vi "InitControlls.vi"(8 "error in (no error)":errorcluster, 11 "Common Refs":T1) -> (0 "error out":errorcluster)   [LabVIEW 2018]
uses:
  TypeDefs/Refs_Common.ctl
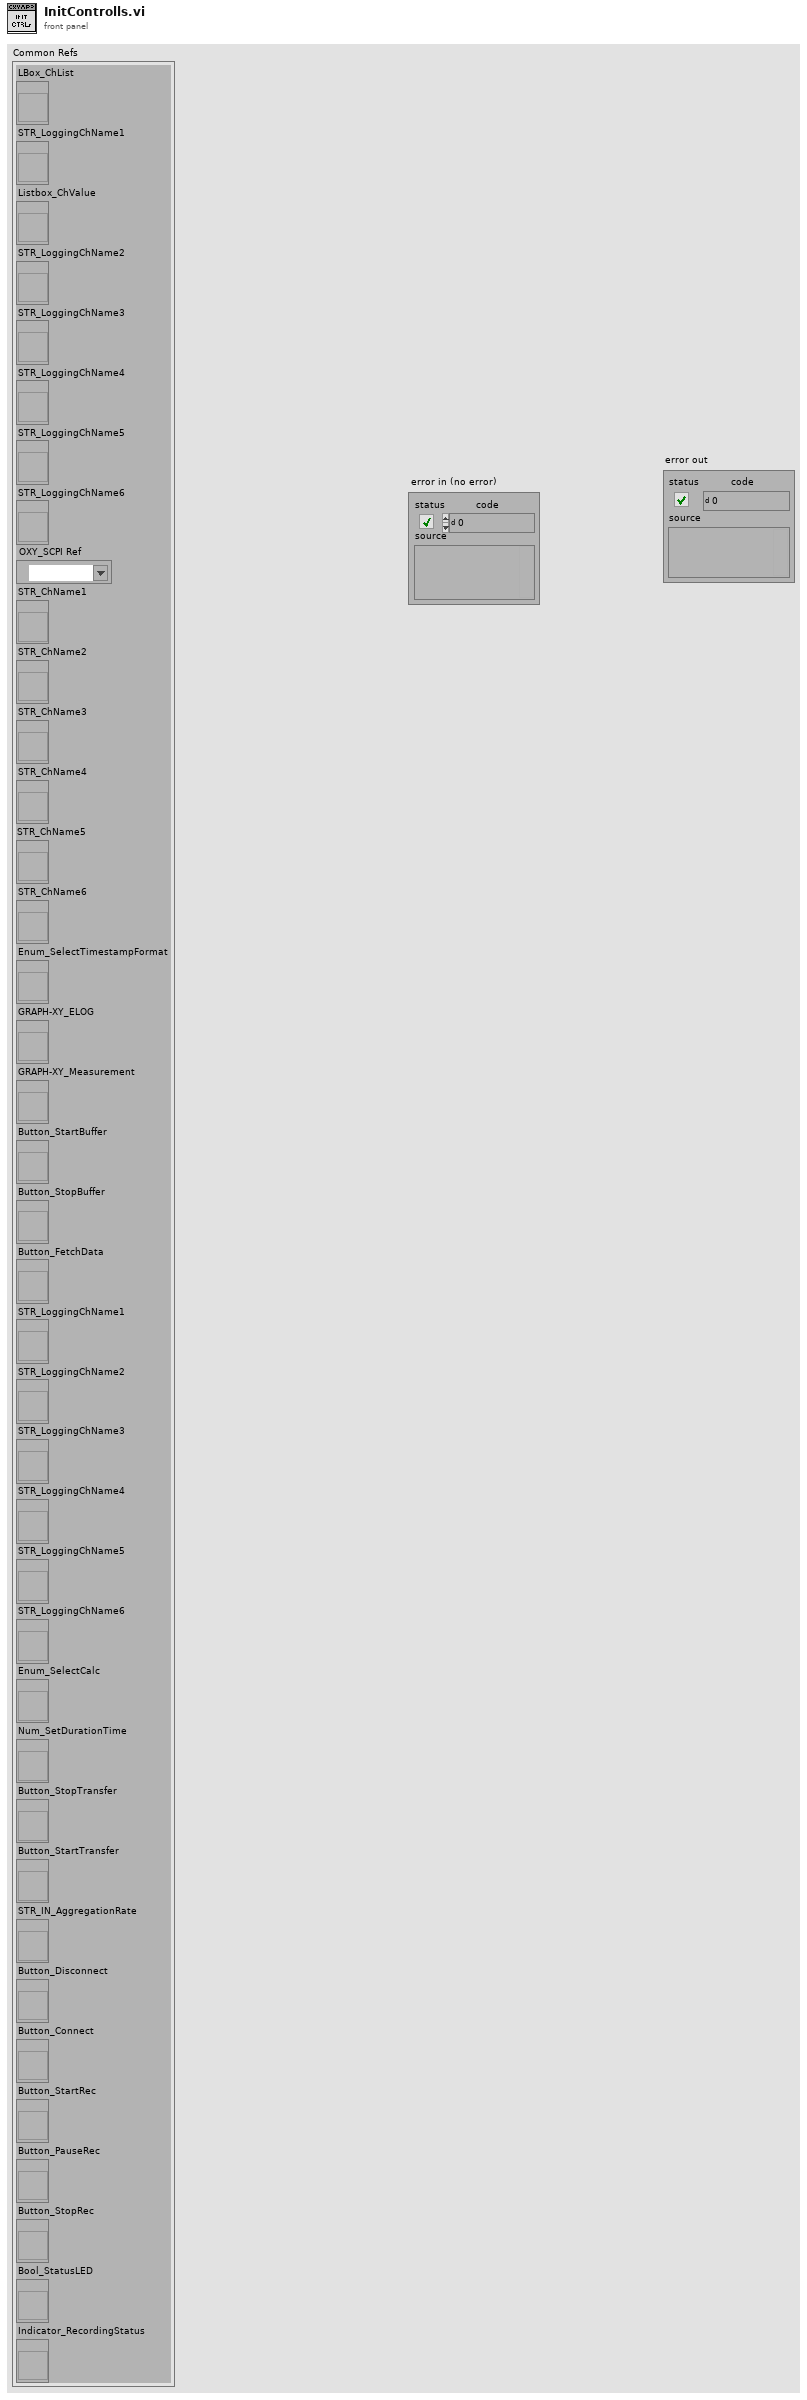
[diagram p1: front panel]
types:
  T1 = typedef "Refs_Common.ctl" = cluster{"LBox_ChList":refnum<vi>, "STR_LoggingChName1":refnum<vi>, "Listbox_ChValue":refnum<vi>, "STR_LoggingChName2":refnum<vi>, "STR_LoggingChName3":refnum<vi>, "STR_LoggingChName4":refnum<vi>, "STR_LoggingChName5":refnum<vi>, "STR_LoggingChName6":refnum<vi>, "OXY_SCPI Ref":refnum<visa-resource-name>, "STR_ChName1":refnum<vi>, "STR_ChName2":refnum<vi>, "STR_ChName3":refnum<vi>, "STR_ChName4":refnum<vi>, "STR_ChName5":refnum<vi>, "STR_ChName6":refnum<vi>, "Enum_SelectTimestampFormat":refnum<vi>, "GRAPH-XY_ELOG":refnum<vi>, "GRAPH-XY_Measurement":refnum<vi>, "Button_StartBuffer":refnum<vi>, "Button_StopBuffer":refnum<vi>, "Button_FetchData":refnum<vi>, "STR_LoggingChName1":refnum<vi>, "STR_LoggingChName2":refnum<vi>, "STR_LoggingChName3":refnum<vi>, "STR_LoggingChName4":refnum<vi>, "STR_LoggingChName5":refnum<vi>, "STR_LoggingChName6":refnum<vi>, "Enum_SelectCalc":refnum<vi>, "Num_SetDurationTime":refnum<vi>, "Button_StopTransfer":refnum<vi>, "Button_StartTransfer":refnum<vi>, "STR_IN_AggregationRate":refnum<vi>, "Button_Disconnect":refnum<vi>, "Button_Connect":refnum<vi>, "Button_StartRec":refnum<vi>, "Button_PauseRec":refnum<vi>, "Button_StopRec":refnum<vi>, "Bool_StatusLED":refnum<vi>, "Indicator_RecordingStatus":refnum<vi>}
  T2 = enum8{"Enabled", "Disabled", "Disabled and Grayed Out"}
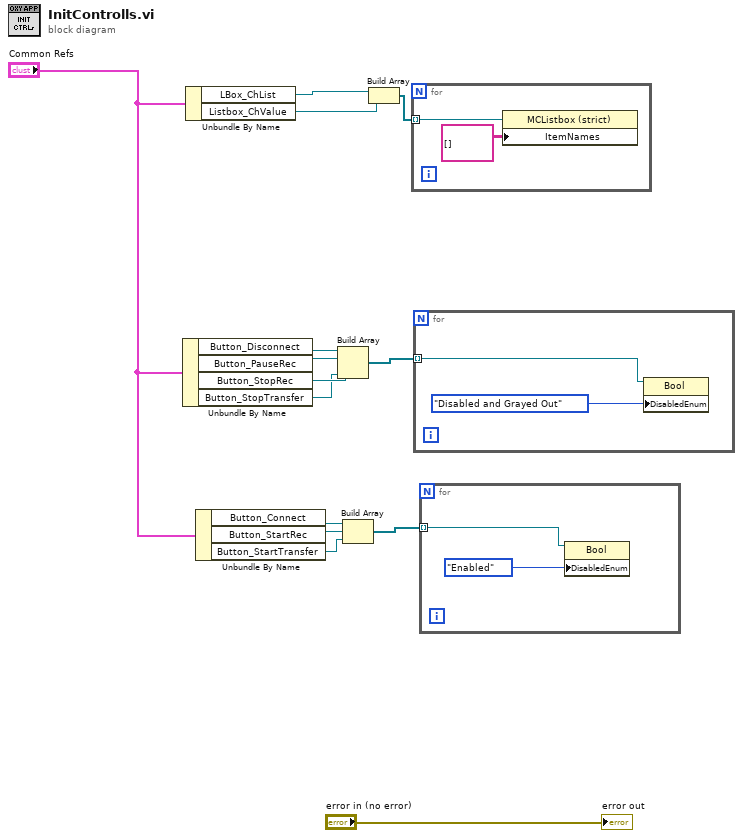
[diagram p0: block diagram]
diagram:
  n1 = Unbundle By Name("Common Refs") -> ("Button_Disconnect"=w10:refnum<vi>, "Button_PauseRec"=w9:refnum<vi>, "Button_StopRec"=w8:refnum<vi>, "Button_StopTransfer"=w1:refnum<vi>)
  n2 = Unbundle By Name("Common Refs") -> ("LBox_ChList"=w12:refnum<vi>, "Listbox_ChValue"=w13:refnum<vi>)
  n3 = Unbundle By Name("Common Refs") -> ("Button_Connect"=w6:refnum<vi>, "Button_StartRec"=w5:refnum<vi>, "Button_StartTransfer"=w2:refnum<vi>)
  n4 = Build Array(w10, w9, w8, w1) -> (w4:refnum<vi>[])
  n5 = Build Array(w6, w5, w2) -> (w3:refnum<vi>[])
  n6 = Build Array(w12, w13) -> (w14:refnum<vi>[])
  n7 = for {
    tunnel: w14 -> [w16] mode=indexing
    n8 = property class="MCListbox (strict)"(reference=w16, "ItemNames"=string[][] [] ("Item Names")) -> ()  [unwired: 1 in, 2 out]
  }
  n9 = for {
    tunnel: w4 -> [w17] mode=indexing
    n10 = property class="Bool"(reference=w17, "DisabledEnum"=T2."Disabled and Grayed Out" ("Disabled")) -> ()  [unwired: 1 in, 2 out]
  }
  n11 = for {
    tunnel: w3 -> [w19] mode=indexing
    n12 = property class="Bool"(reference=w19, "DisabledEnum"=T2."Enabled" ("Disabled")) -> ()  [unwired: 1 in, 2 out]
  }
  "error out" <- "error in (no error)"
